vi "GetActualCameraParameters.vi"(0 "Refnum in":T1, 11 "error in (no error)":errorcluster) -> (4 "ExposureMode":string, 6 "ExposureValue":string, 8 "GainMode":string, 10 "GainValue":string, 14 "InverseExposureValue":dbl, 15 "error out":errorcluster)   [LabVIEW 2015]
uses:
  <vilib>/userdefined/High Color/IMAQdx.ctl
  <resource>/objmgr/imaqdx.rc
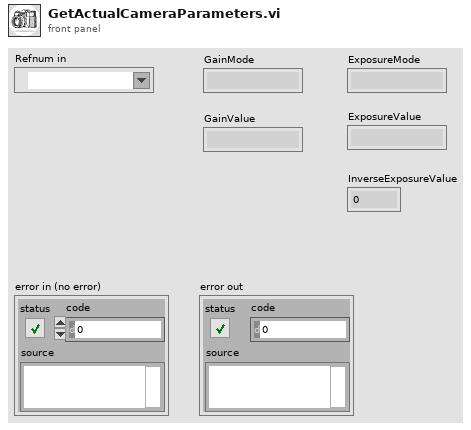
[diagram p1: front panel]
types:
  T1 = typedef "IMAQdx.ctl" = refnum<k21>
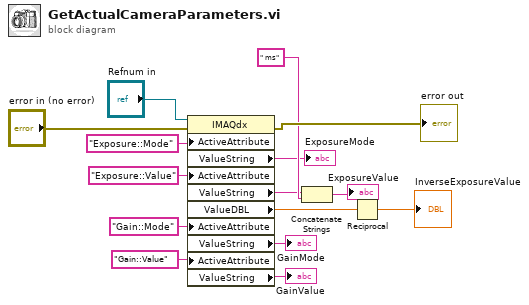
[diagram p0: block diagram]
diagram:
  n1 = property class="IMAQdx"(reference="Refnum in", error in="error in (no error)", "ActiveAttribute"="Exposure::Mode", "ActiveAttribute"="Exposure::Value", "ActiveAttribute"="Gain::Mode", "ActiveAttribute"="Gain::Value") -> (error out=→"error out":errorcluster, "ValueString"=→"ExposureMode":string, "ValueString"=w3:string, "ValueDBL"=w6:dbl, "ValueString"=→"GainMode":string, "ValueString"=→"GainValue":string)  [unwired: 1 out]
  n2 = Concatenate Strings(w3, " ms" ("string")) -> (→"ExposureValue":string)
  n3 = Reciprocal(x=w6) -> (1/x=→"InverseExposureValue":dbl)
